vi "Update Scene Hierarchy.vi"(8 "error in (no error)":errorcluster, 11 "Scene in":refnum<class "Scene.lvclass">) -> (0 "error out":errorcluster)   [LabVIEW 2022 SP3, in "Application.lvlib" / "Scene.lvclass"]
uses:
  Scene.lvclass
  Scene.lvclass/Scene.ctl
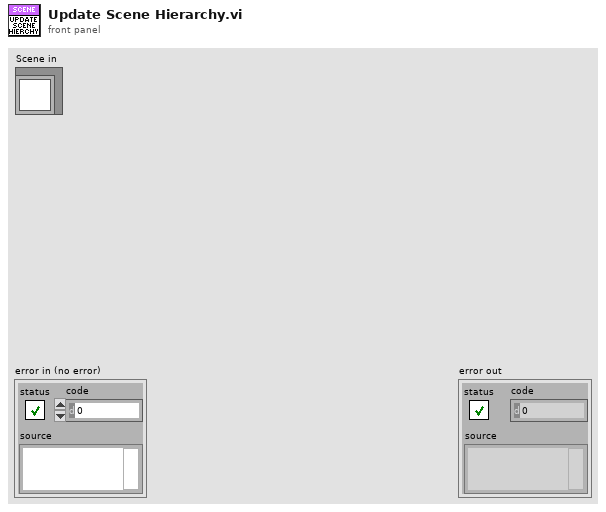
[diagram p1: front panel]
types:
  T1 = typedef "3D.lvlib/Object.ctl" = cluster{"Triangles":T2[], "Diffuse Colour":u32, "Transform":T4, "Name":string}
  T2 = typedef "3D.lvlib/Triangle 3D.ctl" = cluster{"Point 1":T3, "Point 2":T3, "Point 3":T3}
  T3 = typedef "3D.lvlib/Vector 3D.ctl" = cluster{"x":sgl, "y":sgl, "z":sgl}
  T4 = typedef "3D.lvlib/Transform.ctl" = cluster{"Position":T3, "Rotation":T3, "Scale":T3}
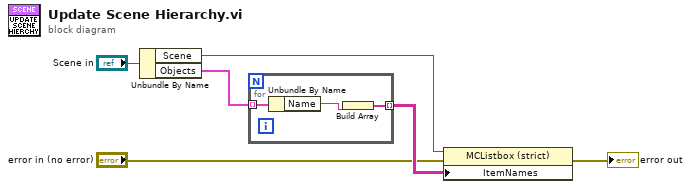
[diagram p0: block diagram]
diagram:
  n1 = Unbundle By Name("Scene in") -> ("Scene"=w5:refnum<vi>, "Objects"=w1:T1[])
  n2 = for {
    tunnel: w1 -> [w9] mode=indexing
    tunnel: [w7] -> w4 mode=indexing
    n3 = Unbundle By Name(w9) -> ("Name"=w8:string)
    n4 = Build Array(w8) -> (w7:string[])
  }
  n5 = property class="MCListbox (strict)"(reference=w5, error in="error in (no error)", "ItemNames"=w4) -> (error out=→"error out":errorcluster)  [unwired: 1 out]
